vi "模拟输出_连续(非可重生成).vi"() -> ()   [LabVIEW 2013]
doc: "This example demonstrates how to output a continuous update waveform."
uses:
  <userlib>/ArtDAQ/_SubVI/ArtDAQ_CreateAOVoltageChan.vi
  <userlib>/ArtDAQ/_SubVI/ArtDAQ_CfgSampClkTiming.vi
  <userlib>/ArtDAQ/_SubVI/ArtDAQ_CfgDigEdgeStartTrig.vi
  <userlib>/ArtDAQ/_SubVI/ArtDAQ_Write Analog DBL NChan NSamp.vi
  <vilib>/Analysis/NI_AALBase.lvlib
panel:
  in  "?":bool
  in  "周期1":dbl=1000.0 format="%#_13g"
  in  "幅值(V)1":dbl=3.0 format="%#_13g"
  in  "周期0":dbl=1000.0 format="%#_13g"
  in  "幅值(V)0":dbl=3.0 format="%#_13g"
  in  "?":enum32{"无触发", "数字边沿触发"}(tab)
  in  "触发源":string="/Dev1/PFI1"
  in  "触发边沿":i32(ring)=10280 items=["上升"=10280, "下降"=10171]
  out "波形图":dbl[][](graph)
  in  "采样速率":dbl=1000.0
  in  "每通道输出点数":i32=4000
  in  "最大值(V)":dbl=10.0
  in  "最小值(V)":dbl=-10.0
  in  "物理通道":string(combo)="Dev1/ao0:1"
  out "错误输出":errorcluster
  # "Channel Parameters"
  # "定时参数"
  # "波形"
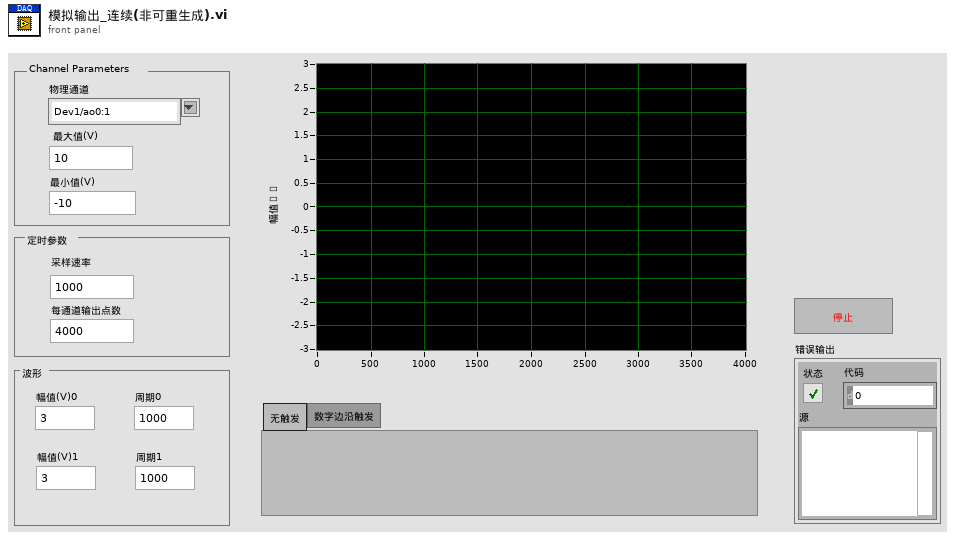
[diagram p1: front panel]
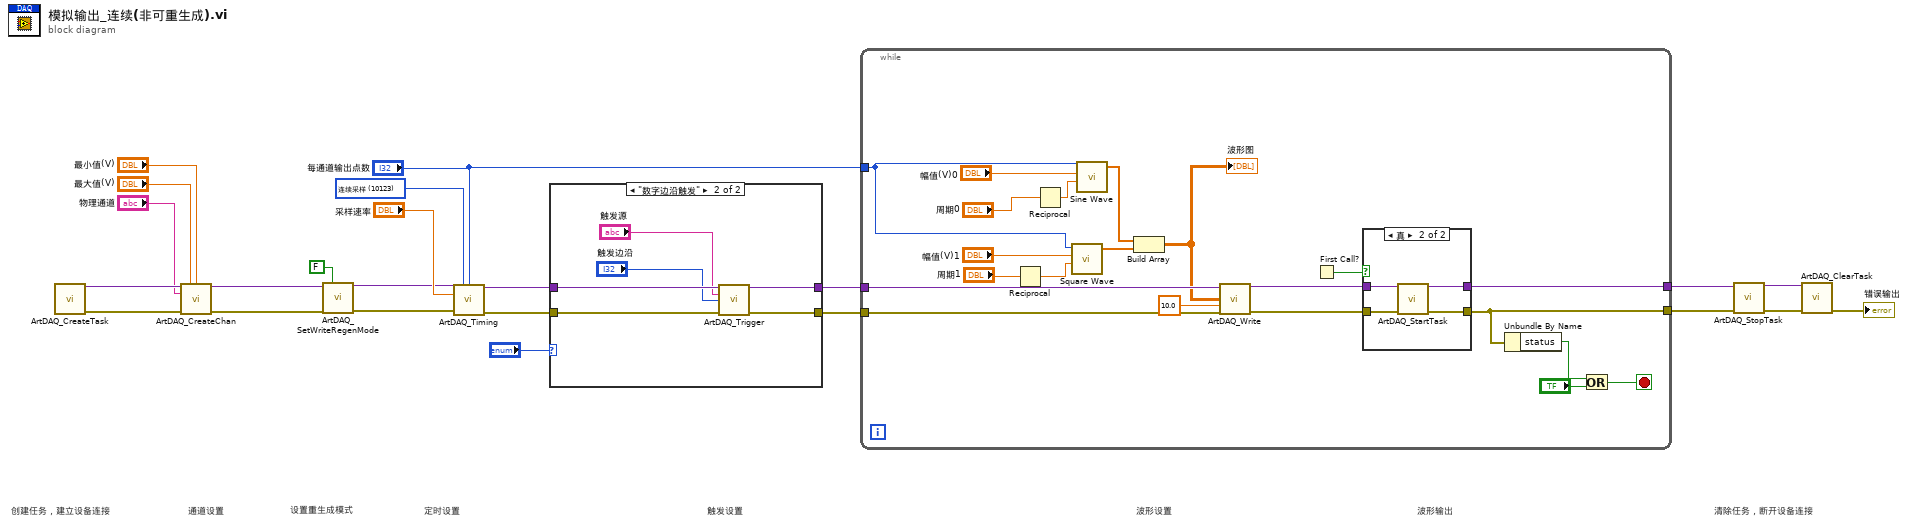
[diagram p0: block diagram]
diagram:
  w14 = 10123 items=["有限点采样"=10178, "连续采样"=10123] ("SampleMode")
  # "设置重生成模式"
  # "清除任务，断开设备连接"
  # "波形输出"
  # "波形设置"
  # "触发设置"
  # "定时设置"
  # "通道设置"
  # "创建任务，建立设备连接"
  n1 = call <userlib>:"ArtDAQ_CreateTask.vi"() -> ("任务句柄"=w23:variant, "错误输出"=w22:errorcluster)  [unwired: 14 in]
  n2 = call-poly <userlib>:"ArtDAQ_CreateChan.vi"("任务句柄"=w23, "最大值"="最大值(V)", "最小值"="最小值(V)", "物理通道"="物理通道", "错误输入"=w22) -> ("任务句柄"=w4:variant, "错误输出"=w6:errorcluster)  [unwired: 9 in]
  n3 = call <userlib>:"ArtDAQ_SetWriteRegenMode.vi"("任务句柄"=w4, "可重生成？"=FALSE ("OverWrite"), "错误输入"=w6) -> ("任务句柄"=w3:variant, "错误输出"=w5:errorcluster)  [unwired: 11 in]
  n4 = call-poly <userlib>:"ArtDAQ_Timing.vi"("任务句柄"=w3, "采样模式"=w14, "每通道采样数"="每通道输出点数", "采样率"="采样速率", "错误输入"=w5) -> ("任务句柄"=w11:variant, "错误输出"=w9:errorcluster)  [unwired: 9 in]
  n5 = case shown="\"数字边沿触发\"" "?" {
    tunnel: w11 -> [w25 w31]
    tunnel: [w25 w30] -> w10
    tunnel: w9 -> [w24 w28]
    tunnel: [w24 w29] -> w8
    frame "无触发", Default {
    }
    frame "数字边沿触发" {
      n6 = call-poly <userlib>:"ArtDAQ_Trigger.vi"("任务句柄"=w31, "触发源"="触发源", "边沿"="触发边沿", "错误输入"=w28) -> ("任务句柄"=w30:variant, "错误输出"=w29:errorcluster)  [unwired: 10 in]
    }
  }
  n7 = while {
    tunnel: [w42] -> w1
    tunnel: [w41] -> w13
    tunnel: "每通道输出点数" -> [w32]
    tunnel: w10 -> [w46]
    tunnel: w8 -> [w45]
    stop <- w40 stop-if-true
    n8 = Reciprocal(x="周期1") -> (1/x=w37:dbl)
    n9 = Reciprocal(x="周期0") -> (1/x=w49:dbl)
    n10 = call <vilib>:"Square Wave.vi"("samples"=w32, "amplitude"="幅值(V)1", "frequency"=w37) -> ("square wave"=w36:dbl[])  [unwired: 3 in, 2 out]
    n11 = call <vilib>:"Sine Wave.vi"("samples"=w32, "amplitude"="幅值(V)0", "frequency"=w49) -> ("sine wave"=w35:dbl[])  [unwired: 2 in, 2 out]
    n12 = Build Array(w35, w36) -> (w34:dbl[][])
    "波形图" <- w34
    n13 = call-poly <userlib>:"ArtDAQ_Write.vi"("任务句柄"=w46, "数据"=w34, "超时s"=10.0 ("Timeout"), "错误输入"=w45) -> ("任务句柄"=w50:variant, "错误输出"=w51:errorcluster)  [unwired: 9 in, 1 out]
    n14 = First Call?() -> (First Call?: T/F=w43:bool)
    n15 = case shown="真" w43 {
      tunnel: w51 -> [w53 w58]
      tunnel: w50 -> [w54 w57]
      tunnel: [w54 w56] -> w42
      tunnel: [w53 w55] -> w41
      frame False {
      }
      frame True {
        n16 = call <userlib>:"ArtDAQ_StartTask.vi"("任务句柄"=w57, "错误输入"=w58) -> ("任务句柄"=w56:variant, "错误输出"=w55:errorcluster)  [unwired: 12 in]
      }
    }
    n17 = Unbundle By Name(w41) -> ("status"=w44:bool)
    n18 = Or(x=w44, y="?") -> (x .or. y?=w40:bool)
  }
  n19 = call <userlib>:"ArtDAQ_StopTask.vi"("任务句柄"=w1, "错误输入"=w13) -> ("任务句柄"=w21:variant, "错误输出"=w20:errorcluster)  [unwired: 12 in]
  n20 = call <userlib>:"ArtDAQ_ClearTask.vi"("任务句柄"=w21, "错误输入"=w20) -> ("错误输出"=→"错误输出":errorcluster)  [unwired: 13 in]
